vi "EXO61.vi"() -> ()   [LabVIEW 2018]
panel:
  in  "Phase 4":dbl
  in  "Phase 3":dbl
  in  "Phase 2":dbl
  in  "Phase 1":dbl
  out "Orang":bool
  out "Rouge":bool
  out "Vert":bool
  in  "stop":bool
  out "Numeric":u32
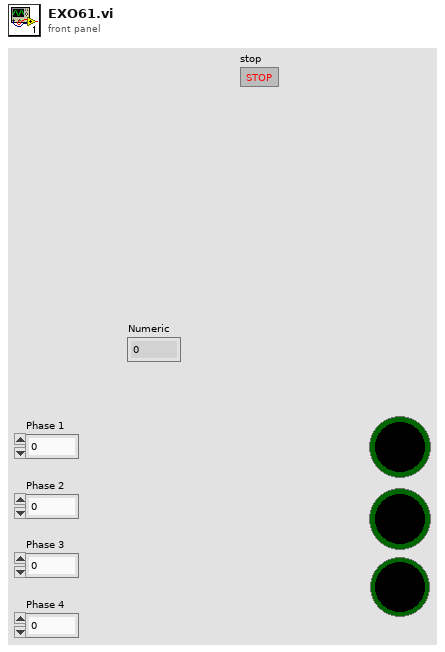
[diagram p1: front panel]
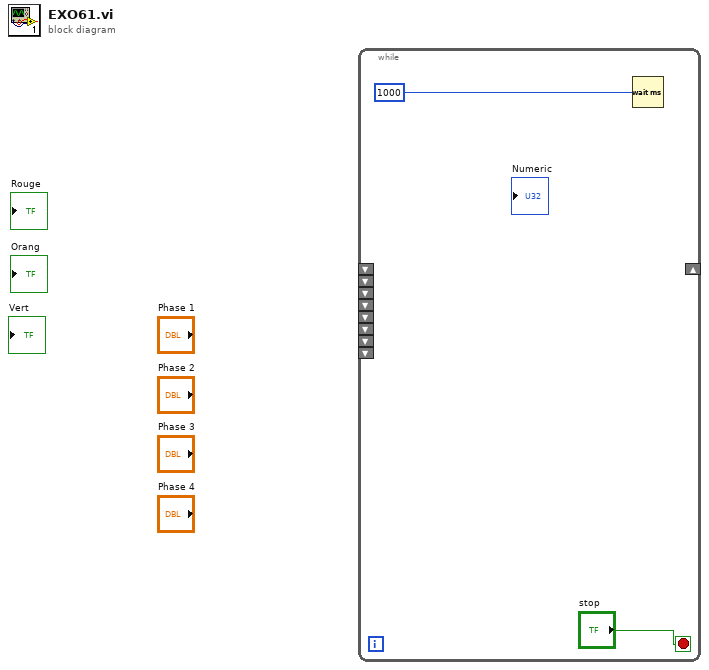
[diagram p0: block diagram]
diagram:
  n1 = while {
    shift-right: _ -> [_]
    shift-left: _ -> [_]
    shift-left: _ -> [_]
    shift-left: _ -> [_]
    shift-left: _ -> [_]
    shift-left: _ -> [_]
    shift-left: _ -> [_]
    shift-left: _ -> [_]
    shift-left: _ -> [_]
    stop <- "stop" stop-if-true
    n2 = Wait (ms)(milliseconds to wait=u32 1000) -> ()  [unwired: 1 out]
  }
